vi "Utility Save or Recall System.vi"(0 "VISA resource name":refnum<visa-resource-name>, 5 "Save/Recall (F: Recal)":bool, 7 "Memory Location (1)":i8=1 min=1 max=101 step=1, 11 "error in (no error)":errorcluster) -> (4 "VISA resource name out":refnum<visa-resource-name>, 15 "error out":errorcluster)   [LabVIEW 2015, in "Chroma ATE 6310.lvlib"]
doc: "This VI stores/recalls settings.\n\nUse this VI to save or recall the present settings from the specified location in memory."
uses:
  <instrlib>/Chroma ATE 6310/Chroma ATE 6310.lvlib
panel:
  # "Save\n\nRecall"
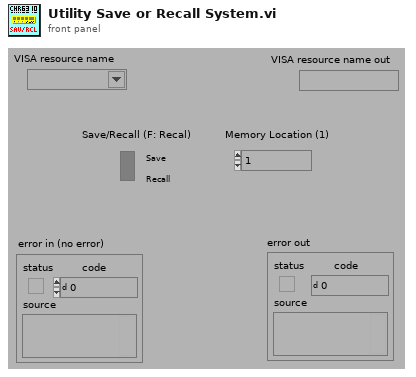
[diagram p1: front panel]
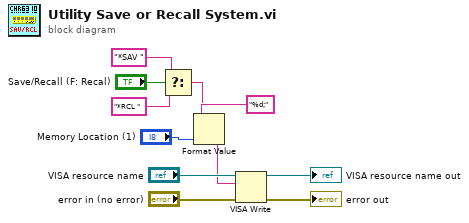
[diagram p0: block diagram]
diagram:
  n1 = Select(t="*SAV ", s="Save/Recall (F: Recal)", f="*RCL ") -> (s? t:f=w7:string)
  n2 = Format Value(string ("")=w7, format string="%d;", value (0)="Memory Location (1)") -> (output string=w1:string)
  n3 = VISA Write(VISA resource name="VISA resource name", write buffer=w1, error in (no error)="error in (no error)") -> (VISA resource name out=→"VISA resource name out":refnum<visa-resource-name>, error out=→"error out":errorcluster)  [unwired: 1 out]
